vi "Populate package files.vi"(0 "Packages Path":path, 11 "error in (no error)":errorcluster) -> (4 "Path Out":path, 6 "Filenames":string[](array[string]), 15 "error out":errorcluster)   [LabVIEW 2021, in "Packager Helpers.lvlib"]
uses:
  Packager Helpers.lvlib
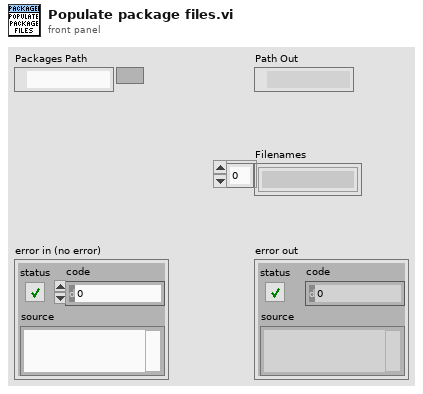
[diagram p1: front panel]
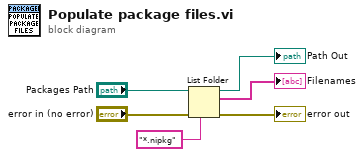
[diagram p0: block diagram]
diagram:
  n1 = List Folder(path="Packages Path", pattern="*.nipkg", error in="error in (no error)") -> (path out=→"Path Out":path, filenames=→"Filenames":string[], error out=→"error out":errorcluster)  [unwired: 1 in, 1 out]
